vi "Reshape Speed Data.vi"(7 "Funct data structure":bool, 9 "Number of time series microscope data frames":u32, 11 "all rows":string[][](array[string])) -> (0 "Averaged RPM speeds array (one speed value per image frame)":dbl[](array[numeric]), 1 "Speed max/min":cluster{"max value":dbl, "min value":dbl}, 2 "Averaged CM/SEC speeds array (one speed value per image frame)":dbl[](array[numeric]), 3 "Speed Data":string[][](array[string]), 4 "Output number of speed points \n(after interpolation)":i32, 5 "Points per frame (fractional)":dbl)   [LabVIEW 2017]
uses:
  Typedefs/HW config states enum.ctl
panel:
  out "# points match":bool
  out "Number of averaged speed points":i32
  out "Number of valid speed points":i32
  out "Original number of points":i32
  out "Fractional index increment\nfor interpolation":dbl
  out "Ideal number of points":i32
  out "Fractional indexes used":dbl[](array[numeric])
  out "Waveform Graph":cluster{"Valid speed data array":dbl[]}[](graph)
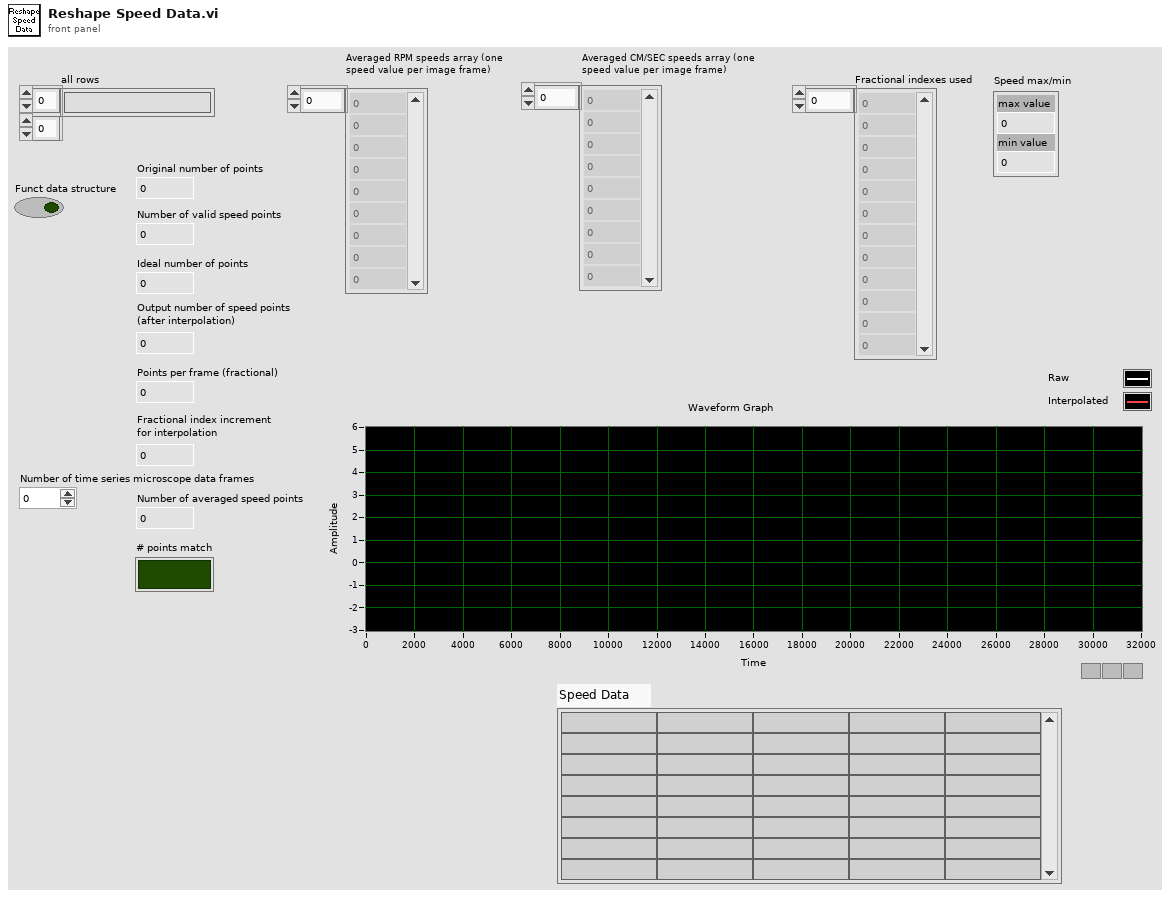
[diagram p1: front panel]
types:
  T1 = typedef "HW config states enum.ctl" = enum16{"Load from file", "Save to file", "Write all", "Read all", "Write XY stage settings", "Write DAQ FPGA settings", "Write Control FPGA settings", "Write Phys Channels", "Clear", "Compare from file"}
  T2 = typedef "Hardware Configuration settings.ctl" = cluster{"Computer MAC address":string, "XY Stage":T3, "Cam VidRec":T4, "Control Sys. HW config":T5, "DAQ FPGA HW Config":cluster{"Target":T6, "input card type":T7}, "DAQmx Chan":T8, "Encoder":T9, "Z Stage config cluster":T10, "Trigger HW config":T11, "Externalise Triggers":bool, "MC Supported":bool, "Laser 1 config cluster":T12, "Prechirper 1 config cluster":T13, "Laser Power Control HW config":T14, "No of AOD":u8, "Dev. PC":bool, "Swap XY on stage":bool, "Axial MC":bool}
  T3 = typedef "XY Stage config cluster.ctl" = cluster{"COM port":refnum<visa-resource-name>, "XY stage available":bool, "Baudrate":i32, "Type":string}
  T4 = typedef "Cam VidRec HW config setup cluster.ctl" = cluster{"DO flag-Video record":tag, "DO flag-Trial start":tag, "VidRec available":bool}
  T5 = typedef "Control Sys HW config cluster.ctl" = cluster{"Control system.FPGA available?":bool, "Control system.FPGA Type":string, "Control system.Network adapter name":string, "Control system.MAC address":string, "Control system.Ethernet Port":u32}
  T6 = typedef "nirio_resource_hc.ctl" = tag
  T7 = typedef "FPGA input type AC-DC.ctl" = enum16{"AC Card", "DC Card"}
  T8 = typedef "DAQmx physical channels cluster.ctl" = cluster{"Pockels AO":tag, "Hard shutter AO":tag, "PMT AOs":tag, "Power meter AI":tag}
  T9 = typedef "Encoder config cluster.ctl" = cluster{"IP address":string, "Port":u16, "Encoder available":bool, "Wheel radius (cm)":dbl, "Encoder Trigger":tag}
  T10 = typedef "Z Stage config cluster.ctl" = cluster{"COM port":refnum<visa-resource-name>, "Z stage available":bool, "Baudrate":i32, "Type":string}
  T11 = typedef "Triggers HW config.ctl" = cluster{"Available Device List":i32, "Device Address":string}
  T12 = typedef "Laser 1 config cluster.ctl" = cluster{"COM port":refnum<visa-resource-name>, "Laser 1 available":bool, "Baud Rate":i32, "Type":string}
  T13 = typedef "PreChirper 1 config cluster.ctl" = cluster{"COM port":refnum<visa-resource-name>, "Prechirper 1 \navailable":bool, "Baud Rate":i32, "Type":string}
  T14 = typedef "Laser Power Control HW config.ctl" = cluster{"Laser Power Control":string, "Laser Power Modulation Control":string}
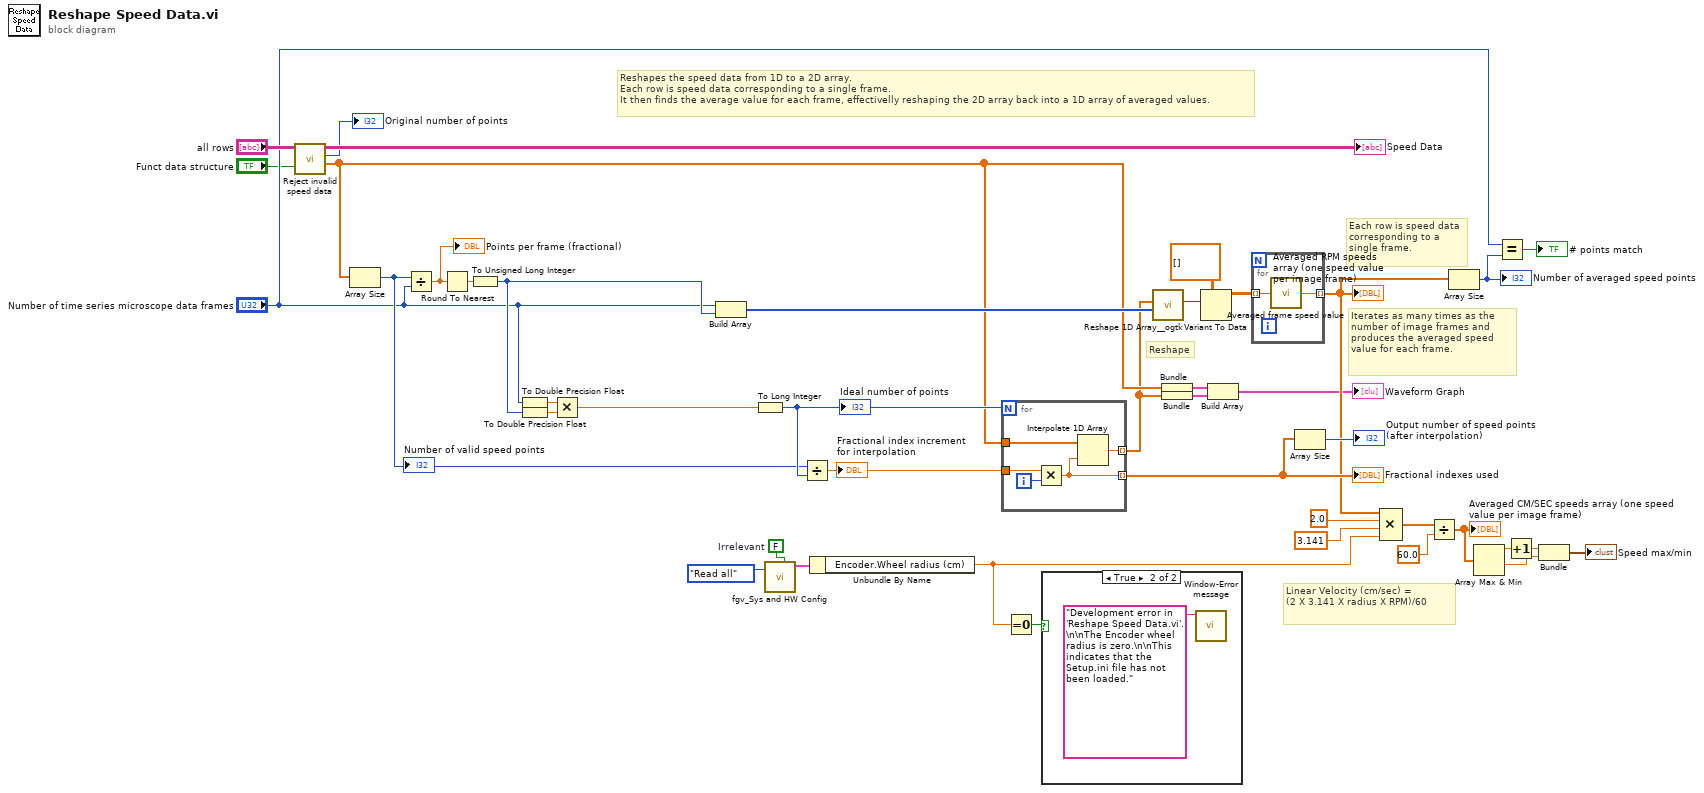
[diagram p0: block diagram]
diagram:
  w1 = FALSE  # Irrelevant
  # "Linear Velocity (cm/sec) = \n(2 X 3.141 X radius X RPM)/60"
  # "Iterates as many times as the number of image frames and produces the averaged speed value for each frame."
  # "Reshape"
  # "Each row is speed data corresponding to a single frame."
  # "Reshapes the speed data from 1D to a 2D array.\nEach row is speed data corresponding to a single frame.\nIt then finds the average value for each frame, effectivelly reshaping the 2D array back into a 1D array of averaged values."
  n1 = call "Reject invalid speed data.vi"("Funct data structure"="Funct data structure", "Spreadsheet data"="all rows") -> ("Valid speed data"=w13:dbl[], "Original number of points"=→"Original number of points":i32, "Valid speed data table"=→"Speed Data":string[][])  [unwired: 7 in]
  n2 = Array Size(array=w13) -> (size(s)=w23:i32)
  "Number of valid speed points" <- w23
  n3 = Divide(x=w23, y="Number of time series microscope data frames") -> (x/y=w35:dbl)
  "Points per frame (fractional)" <- w35
  n4 = Round To Nearest(number=w35) -> (nearest integer value=w37:dbl)
  n5 = To Unsigned Long Integer(number=w37) -> (unsigned 32bit integer=w33:u32)
  n6 = To Double Precision Float(number="Number of time series microscope data frames") -> (double precision float=w21:dbl)
  n7 = To Double Precision Float(number=w33) -> (double precision float=w20:dbl)
  n8 = Multiply(x=w21, y=w20) -> (x*y=w36:dbl)
  n9 = Build Array("Number of time series microscope data frames", w33) -> (w32:u32[])
  n10 = To Long Integer(number=w36) -> (32bit integer=w34:i32)
  "Ideal number of points" <- w34
  n11 = call "fgv_Sys and HW Config.vi"("Standalone viewer initialisation?"=w1, "Function"=HW_config_states_enum."Read all") -> ("Hardware Configuration OUT"=w4:T2)  [unwired: 7 in, 2 out]
  n12 = Divide(x=w23, y=w34) -> (x/y=w38:dbl)
  "Fractional index increment\nfor interpolation" <- w38
  n13 = Unbundle By Name(w4) -> ("Encoder.Wheel radius (cm)"=w3:dbl)
  n14 = for {
    N: w34 -> [_]
    tunnel: w38 -> [w45]
    tunnel: w13 -> [w47]
    tunnel: [w44] -> w12 mode=indexing
    tunnel: [w43] -> w31 mode=indexing
    i -> [w46]
    n15 = Multiply(x=w45, y=w46) -> (x*y=w43:dbl)
    n16 = Interpolate 1D Array(1:w43, 2:w47) -> (0:w44:dbl)
  }
  "Fractional indexes used" <- w31
  n17 = Equal To 0?(x=w3) -> (x = 0?=w2:bool)
  n18 = case shown="True" w2 {
    frame False {
    }
    frame True {
      n19 = call "Window-Error message.vi"("Message"="Development error in 'Reshape Speed Data.vi'.\n\nThe Encoder wheel radius is zero.\n\nThis indicates that the Setup.ini file has not been loaded.") -> ()  [unwired: 10 in, 1 out]
    }
  }
  n20 = call <userlib>:"Reshape 1D Array__ogtk.vi"("Size(s)"=w32, "1D Array"=w12) -> ("Reshaped VArray"=w41:variant)  [unwired: 8 in, 1 out]
  n21 = Bundle("Valid speed data"=w13) -> (w11:cluster{"Valid speed data":dbl[]})  [unwired: 1 in]
  n22 = Bundle(w12) -> (w10:cluster{dbl[]})  [unwired: 1 in]
  n23 = Variant To Data(type=dbl[][] [] ("number"), Variant=w41) -> (data=w27:dbl[][])  [unwired: 1 in, 1 out]
  n24 = Build Array(w11, w10) -> (→"Waveform Graph":cluster{"Valid speed data":dbl[]}[])
  n25 = for {
    tunnel: w27 -> [w50] mode=indexing
    tunnel: [w49] -> w18 mode=indexing
    n26 = call "Averaged frame speed value.vi"("Reshaped speed data array"=w50) -> ("Average value"=w49:dbl)
  }
  "Averaged RPM speeds array (one speed value per image frame)" <- w18
  n27 = Array Size(array=w31) -> (size(s)=→"Output number of speed points \n(after interpolation)":i32)
  n28 = Compound Arithmetic op=MULTIPLY(w18, 2.0 ("Fractional index increment\nfor interpolation"), 3.141 ("Fractional index increment\nfor interpolation"), w3) -> (w15:dbl[])
  n29 = Divide(x=w15, y=60.0 ("Fractional index increment\nfor interpolation")) -> (x/y=w7:dbl[])
  "Averaged CM/SEC speeds array (one speed value per image frame)" <- w7
  n30 = Array Size(array=w18) -> (size(s)=w26:i32)
  "Number of averaged speed points" <- w26
  n31 = Array Max & Min(array=w7) -> (max value=w8:dbl, min value=w40:dbl)  [unwired: 2 out]
  n32 = Equal?(x="Number of time series microscope data frames", y=w26) -> (x = y?=→"# points match":bool)
  n33 = Increment(x=w8) -> (x+1=w6:dbl)
  n34 = Bundle(w6, w40) -> (→"Speed max/min":cluster{dbl, dbl})  [unwired: 1 in]
